vi "Untitled 1.vi"() -> ()   [LabVIEW 2015]
panel:
  out "Meter":dbl(knob) scale=0.0..10.0
  out "PRND":string
  out "Speed2":i16 format="%3.0f"
  out "Boolean 2":bool
  out "SPEED":dbl(knob) scale=0.0..200.0 scale format="%_2p"
  out "Boolean":bool
  out "apv 16":bool
  out "apv 15":bool
  out "apv 14":bool
  out "apv 13":bool
  out "apv 12":bool
  out "apv 11":bool
  out "apv 10":bool
  out "apv 9":bool
  out "apv 8":bool
  out "apv 7":bool
  out "apv 6":bool
  out "apv 5":bool
  out "apv 4":bool
  out "apv 3":bool
  out "apv 2":bool
  out "apv 1":bool
  # "km/h"
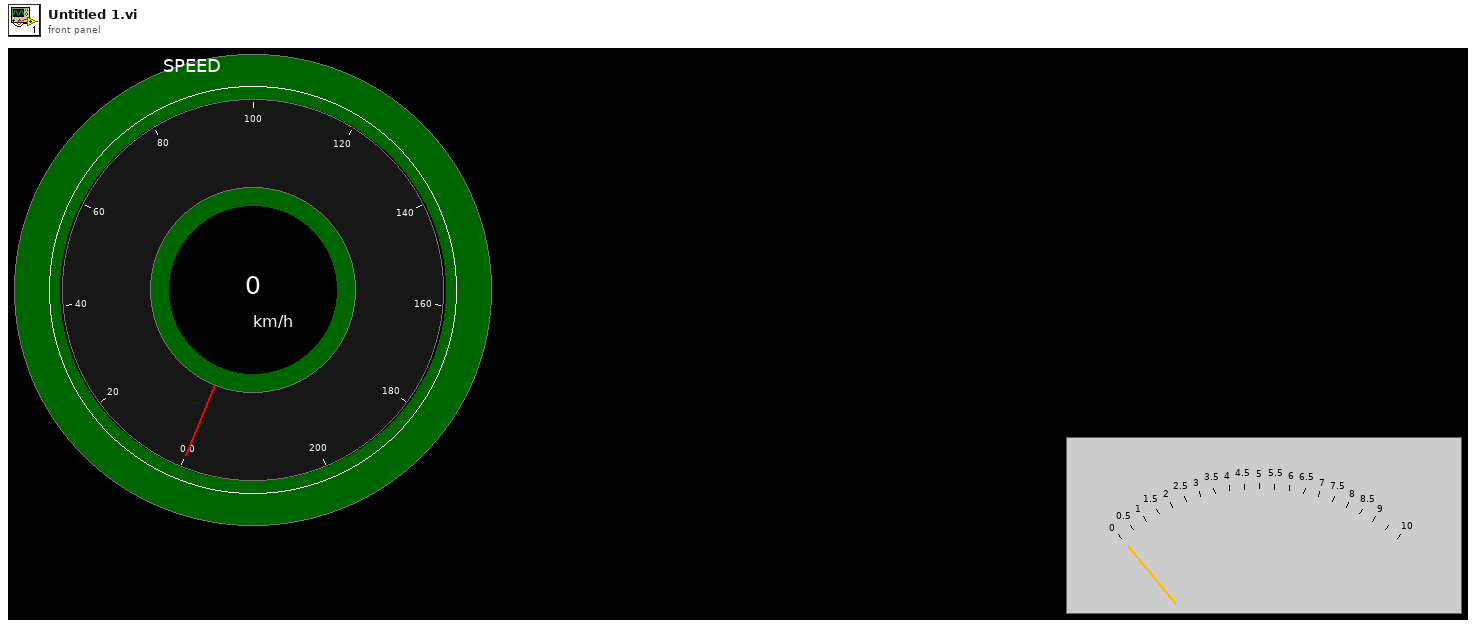
[diagram p1: front panel]
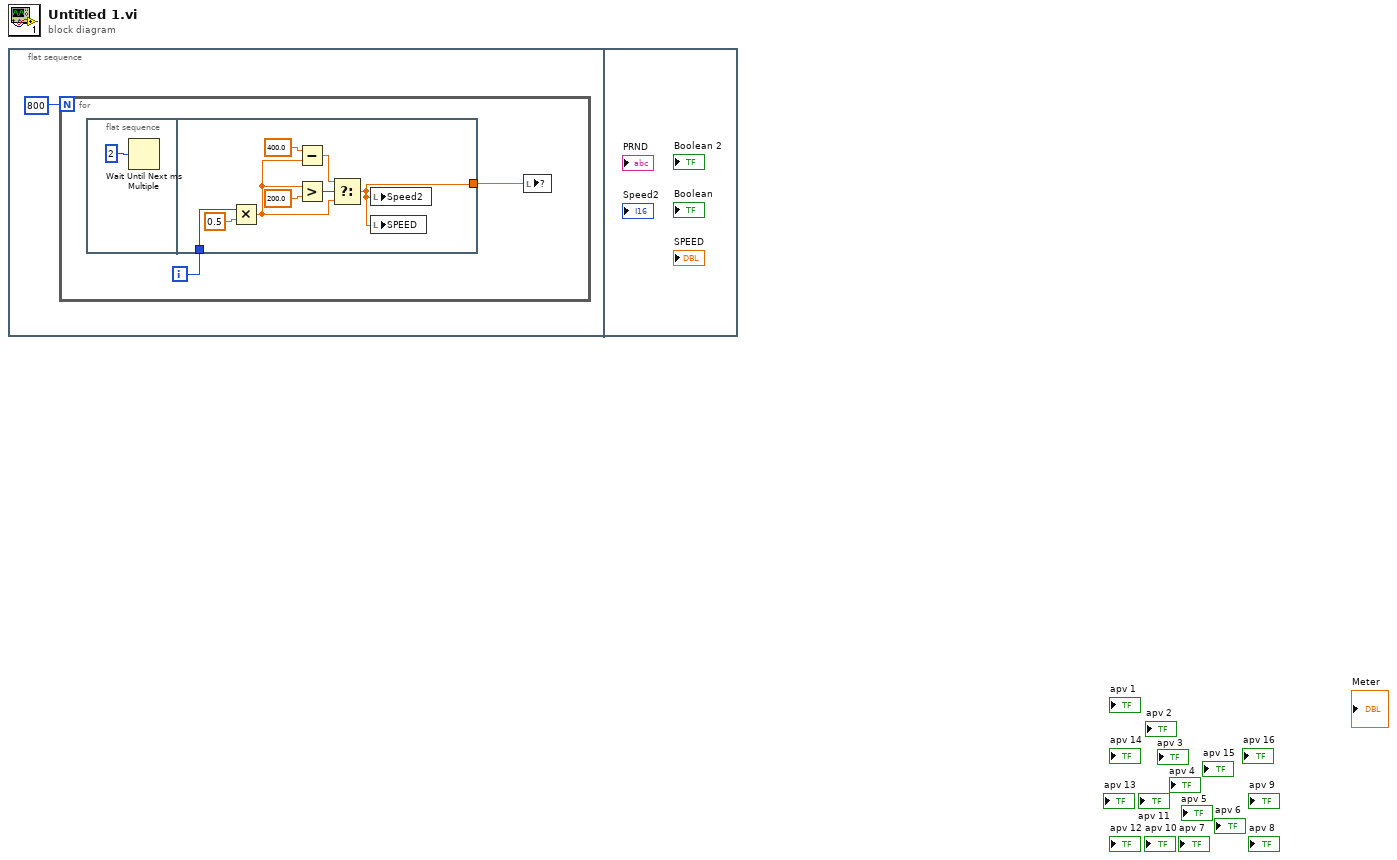
[diagram p0: block diagram]
diagram:
  n1 = flat-sequence {
    frame #0 {
      n2 = for {
        N: 800 -> [_]
        i -> [w3]
        n3 = flat-sequence {
          tunnel: w3 -> [w12]
          tunnel: [w5] -> w2
          frame #0 {
            n4 = Wait Until Next ms Multiple(millisecond multiple=u32 2) -> ()  [unwired: 1 out]
          }
          frame #1 {
            n5 = Multiply(x=w12, y=0.5) -> (x*y=w6:dbl)
            n6 = Subtract(x=400.0, y=w6) -> (x-y=w7:dbl)
            n7 = Greater?(x=w6, y=200.0) -> (0:w9:bool)
            n8 = Select(t=w7, s=w9, f=w6) -> (s? t:f=w5:dbl)
            n9 = local write "Speed2"(w5) -> ()
            n10 = local write "SPEED"(w5) -> ()
          }
        }
        n11 = local write item#-1(w2) -> ()
      }
    }
    frame #1 {
    }
  }
